vi "Review3.vi"() -> ()   [LabVIEW 2018]
panel:
  in  "전체중지":bool
  in  "탭 컨트롤":enum32{"숫자 추가 1", "숫자 추가 2", "구구단", "알람 1"}(tab)
  in  "추가":bool
  in  "정지":bool
  out "배열 2":i32[](array[numeric])
  in  "추가 숫자":i32
  in  "추가 숫자 2":i32
  out "배열 3":i32[](array[numeric])
  in  "추가 2":bool
  out "구구단":i32[][](array[numeric])
  in  "활성화":bool
  in  "타임스탬프":timestamp
  out "불리언":bool
  out "현재 시각":timestamp
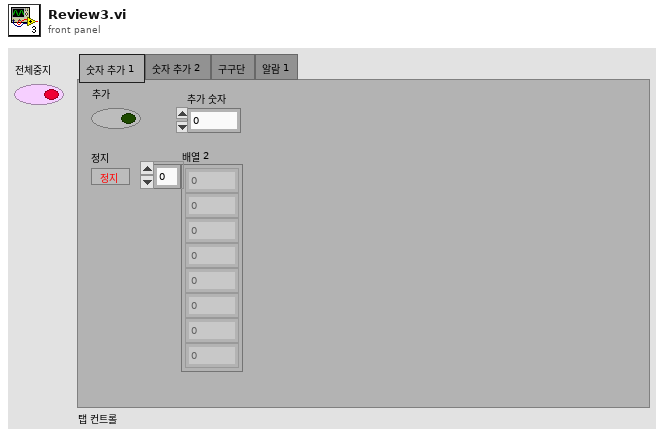
[diagram p1: front panel]
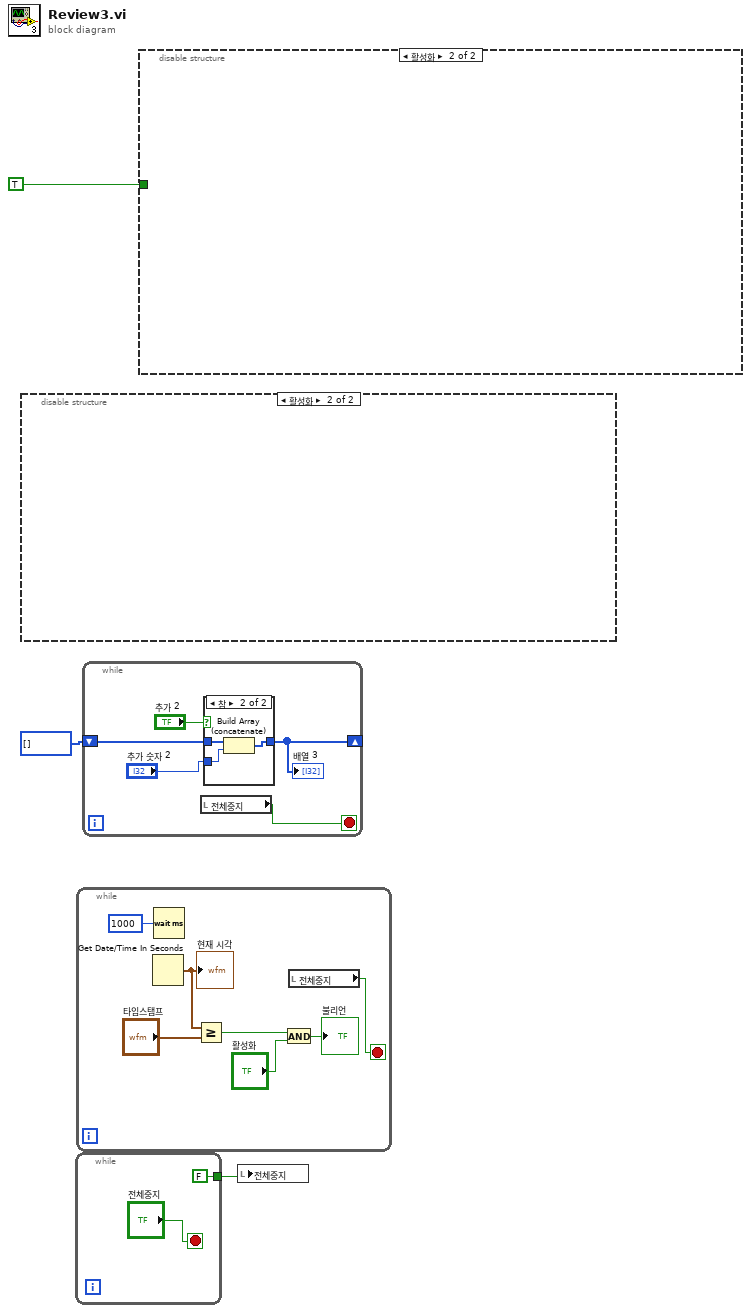
[diagram p0: block diagram]
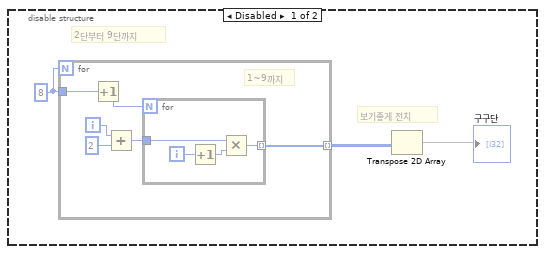
[diagram p3: hidden frame]
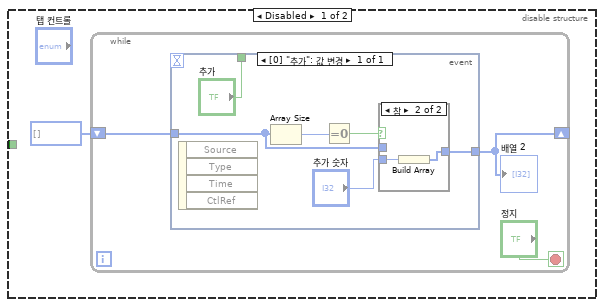
[diagram p4: hidden frame]
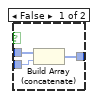
[diagram p5: hidden frame]
diagram:
  n1 = disable-structure shown="활성화" {
    frame Disabled {
      w6 = 8
      # "보기좋게 전치"
      # "2단부터 9단까지"
      n2 = for {
        N: w6 -> [_]
        tunnel: w6 -> [w10]
        tunnel: [w8] -> w5 mode=indexing
        i -> [w11]
        # "1~9까지"
        n3 = Increment(x=w10) -> (x+1=w9:i32)
        n4 = Add(x=w11, y=2) -> (x+y=w7:i32)
        n5 = for {
          N: w9 -> [_]
          tunnel: [w13] -> w8 mode=indexing
          tunnel: w7 -> [w15]
          i -> [w16]
          n6 = Increment(x=w16) -> (x+1=w14:i32)
          n7 = Multiply(x=w15, y=w14) -> (x*y=w13:i32)
        }
      }
      n8 = Transpose 2D Array(2D array=w5) -> (transposed array=→"구구단":i32[][])
    }
    frame Enabled {
    }
  }
  n9 = while {
    tunnel: [FALSE] -> w1
    stop <- "전체중지" stop-if-true
  }
  n10 = while {
    stop <- w20 stop-if-true
    n11 = Get Date/Time In Seconds() -> (seconds since 1Jan1904=w24:timestamp)
    "현재 시각" <- w24
    n12 = Wait (ms)(milliseconds to wait=u32 1000 ("대기 시간 (ms)")) -> ()  [unwired: 1 out]
    n13 = Greater Or Equal?(x=w24, y="타임스탬프") -> (x >= y?=w22:bool)
    n14 = And(x=w22, y="활성화") -> (x .and. y?=→"불리언":bool)
    n15 = local read "전체중지"() -> (w20:bool)
  }
  n16 = while {
    shift-right: [w27] -> _
    shift-left: i32[] [] -> [w28]
    stop <- w26 stop-if-true
    n17 = local read "전체중지"() -> (w26:bool)
    n18 = case shown="참" "추가 2" {
      tunnel: "추가 숫자 2" -> [_ w34]
      tunnel: w28 -> [w31 w33]
      tunnel: [w31 w32] -> w27
      frame False {
      }
      frame True {
        n19 = Build Array (concatenate)(w33, w34) -> (w32:i32[])
      }
    }
    "배열 3" <- w27
  }
  n20 = disable-structure shown="활성화" {
    disable-tunnel: TRUE -> [_ _]
    frame Disabled {
      n21 = while {
        shift-right: [w37] -> _
        shift-left: i32[] [] -> [w36]
        stop <- "정지" stop-if-true
        n22 = event shown="[0] \"추가\": 값 변경" {
          selector: _ -> [_]
          dyn-events: _ -> [_]
          timeout: _ -> [_]
          tunnel: [w44] -> w37
          tunnel: w36 -> [w41]
          tunnel: ["추가"] -> _
          event "추가": Value Change {
            n23 = event-data() -> ()  [unwired: 1 in, 4 out]
            n24 = Array Size(array=w41) -> (size(s)=w42:i32)
            n25 = Equal To 0?(x=w42) -> (x = 0?=w43:bool)
            n26 = case shown="참" w43 {
              tunnel: [w45 w49] -> w44
              tunnel: w41 -> [w47 _]
              tunnel: "추가 숫자" -> [w46 w48]
              frame False {
                n27 = Build Array (concatenate)(w47, w46) -> (w45:i32[])
              }
              frame True {
                n28 = Build Array(w48) -> (w49:i32[])
              }
            }
          }
        }
        "배열 2" <- w37
      }
    }
    frame Enabled {
    }
  }
  n29 = local write "전체중지"(w1) -> ()
